vi "Load Configuration.vi"(8 "error in":errorcluster, 10 "Module Name":string, 11 "Module Data In":refnum<class "Rename.lvclass">) -> (0 "error out":errorcluster, 3 "Module Data Out":refnum<class "Rename.lvclass">)   [LabVIEW 2015, in "Generic Module Library.lvlib" / "Template G_Module.lvlib"]
uses:
  Template G_Module.lvlib
  <vilib>/Utility/xml.llb/Read From XML File(string).vi
  Module Class/Rename.lvclass
panel:
  out "XML Config String":string
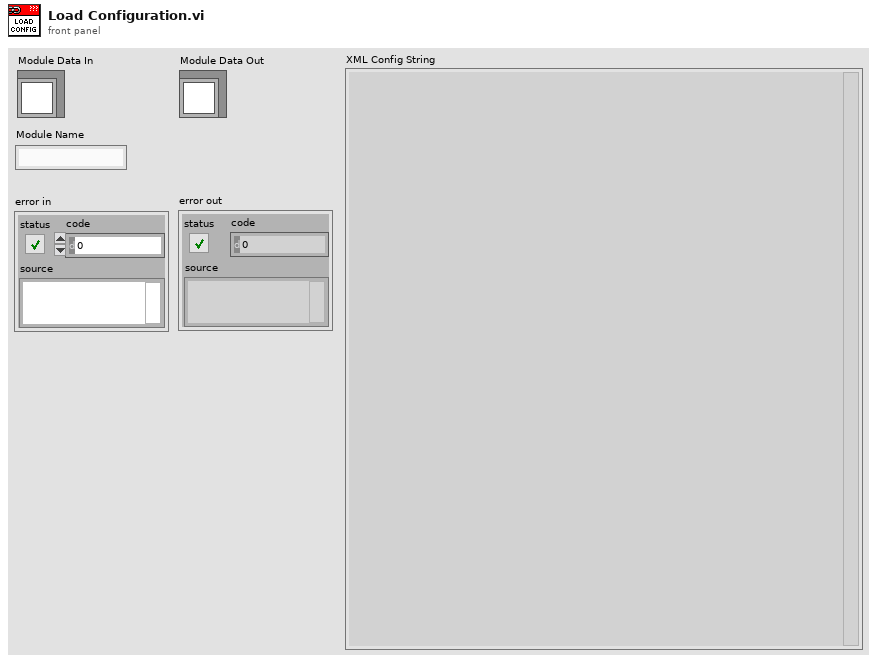
[diagram p1: front panel]
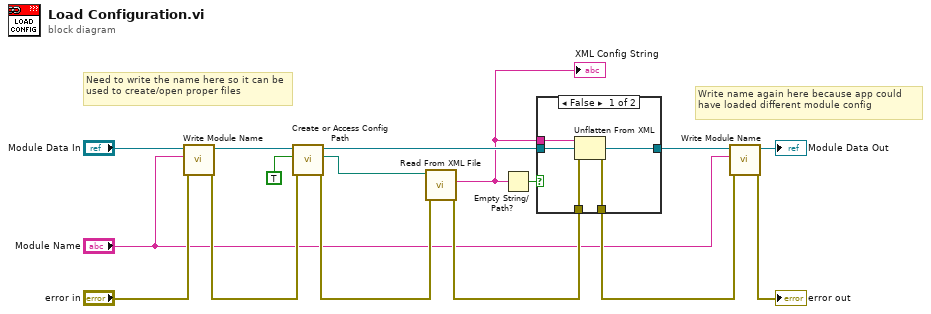
[diagram p0: block diagram]
diagram:
  # "Write name again here because app could have loaded different module config"
  # "Need to write the name here so it can be used to create/open proper files"
  n1 = call-dynamic "Write Module Name.vi"("error in (no error)"="error in", "Module Name"="Module Name", "Rename in"="Module Data In") -> ("error out"=w6:errorcluster, "Rename out"=w8:refnum<class "Rename.lvclass">)  [unwired: 7 in]
  n2 = call "Create or Access Config Path.vi"("error in"=w6, "Check/Build Folders?"=TRUE, "Module Data"=w8) -> ("error out"=w13:errorcluster, "Config File Path"=w15:path, "Module Data"=w14:refnum<class "Rename.lvclass">)  [unwired: 6 in]
  n3 = call-poly <vilib>:"Read From XML File.vi"("error in (no error)"=w13, "XML File Path"=w15) -> ("error out"=w12:errorcluster, "XML Elements"=w10:string)  [unwired: 7 in, 1 out]
  "XML Config String" <- w10
  n4 = Empty String/Path?(string/path=w10) -> (empty?=w11:bool)
  n5 = case shown="False" w11 {
    tunnel: w10 -> [w21 _]
    tunnel: [w20 w23] -> w3
    tunnel: w14 -> [w19 w22]
    tunnel: [w18 w22] -> w5
    tunnel: w12 -> [w17 w23]
    frame False {
      n6 = Unflatten From XML(xml string=w21, type=w19, error in (no error)=w17) -> (value=w18:refnum<class "Rename.lvclass">, error out=w20:errorcluster)
    }
    frame True {
    }
  }
  n7 = call-dynamic "Write Module Name.vi"("error in (no error)"=w3, "Module Name"="Module Name", "Rename in"=w5) -> ("error out"=→"error out":errorcluster, "Rename out"=→"Module Data Out":refnum<class "Rename.lvclass">)  [unwired: 7 in]
